vi "Decode HydroHarp v1 TT Data.vi"(8 "oflcorr_in":u64, 11 "rawbits":u32) -> (0 "oflcorr_out":u64, 1 "channel":u8, 3 "truetime":u64, 4 "markercode":u32)   [LabVIEW 2021, in "PTU Files.lvlib"]
uses:
  PTU Files.lvlib
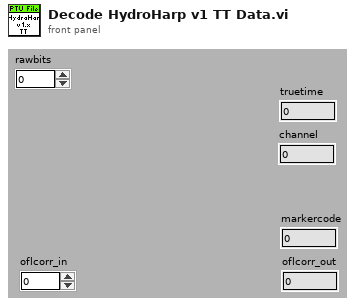
[diagram p1: front panel]
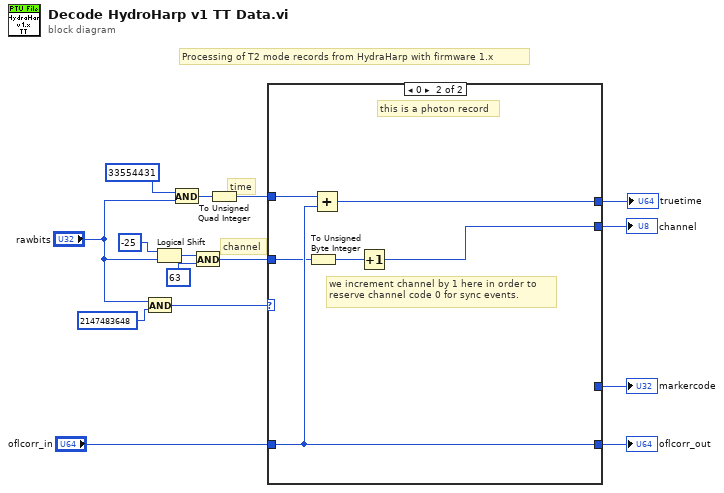
[diagram p0: block diagram]
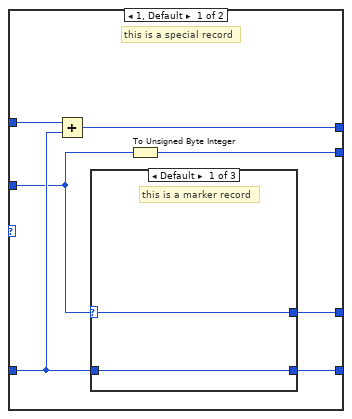
[diagram p2: hidden frame]
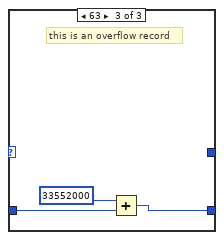
[diagram p4: hidden frame]
diagram:
  # "Processing of T2 mode records from HydraHarp with firmware 1.x"
  # "channel"
  # "time"
  n1 = And(x="rawbits", y=u32 2147483648 ("x")) -> (x .and. y?=w2:u32)
  n2 = Logical Shift(y=-25, x="rawbits") -> (x << y=w12:u32)
  n3 = And(x=u32 33554431, y="rawbits") -> (x .and. y?=w8:u32)
  n4 = And(x=w12, y=u32 63 ("x")) -> (x .and. y?=w1:u32)
  n5 = To Unsigned Quad Integer(1:w8) -> (0:w3:u64)
  n6 = case shown="0" w2 {
    tunnel: w3 -> [w19 w34]
    tunnel: "oflcorr_in" -> [w20 w32]
    tunnel: [w22 w32] -> w10
    tunnel: [w21 _] -> w11
    tunnel: [w18 w33] -> w14
    tunnel: [w16 w30] -> w15
    tunnel: w1 -> [w17 w31]
    frame 1, Default {
      # "this is a special record"
      n7 = Add(x=w19, y=w20) -> (x+y=w18:u64)
      n8 = case shown="Default" w17 {
        selector: w17 -> [w23 _ _]
        tunnel: w20 -> [w24 w25 w28]
        tunnel: [w24 w25 w27] -> w22
        tunnel: [w23 _ _] -> w21
        frame Default {
          # "this is a marker record"
        }
        frame 0 {
          # "this is a sync record"
        }
        frame 63 {
          # "this is an overflow record"
          n9 = Add(x=u64 33552000, y=w28) -> (x+y=w27:u64)
        }
      }
      n10 = To Unsigned Byte Integer(number=w17) -> (unsigned 8bit integer=w16:u8)
    }
    frame 0 {
      # "we increment channel by 1 here in order to\nreserve channel code 0 for sync events."
      # "this is a photon record"
      n11 = To Unsigned Byte Integer(number=w31) -> (unsigned 8bit integer=w29:u8)
      n12 = Add(x=w34, y=w32) -> (x+y=w33:u64)
      n13 = Increment(x=w29) -> (x+1=w30:u8)
    }
  }
  "channel" <- w15
  "truetime" <- w14
  "markercode" <- w11
  "oflcorr_out" <- w10
